vi "Main.vi"() -> ()   [LabVIEW 2011]
panel:
  out "Path":path
  out "Time Stamp":timestamp
  out "Waveform Chart":dbl[](graph)
  out "Error Source Information":string
  in  "stop":bool
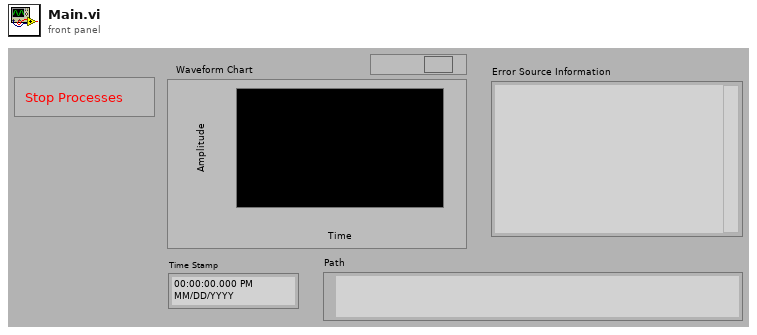
[diagram p1: front panel]
types:
  T1 = cluster{"Data":refnum<user-event>, "Error":refnum<user-event>}
  T2 = cluster{"File Logging":refnum<user-event>, "Error":refnum<user-event>}
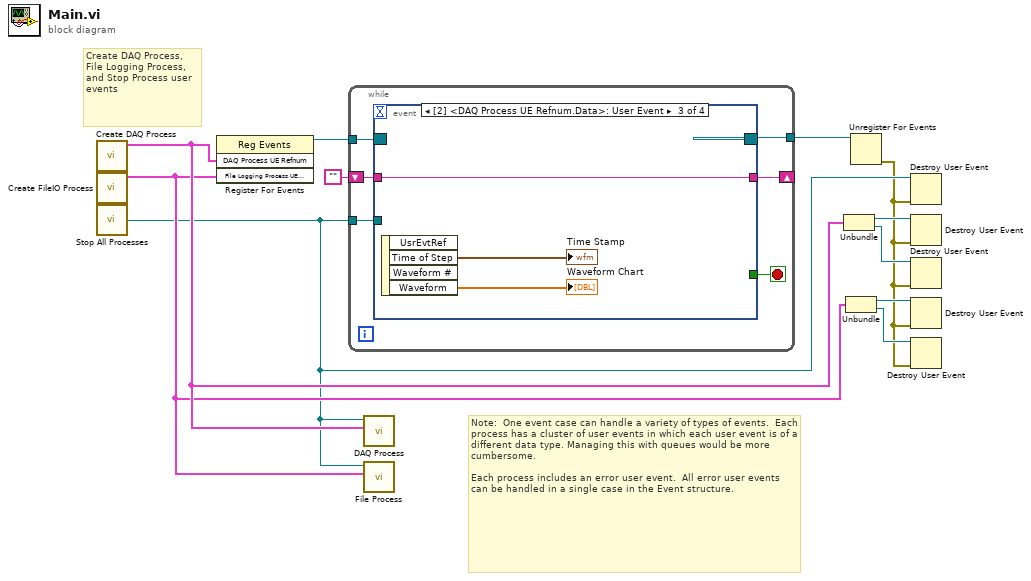
[diagram p0: block diagram]
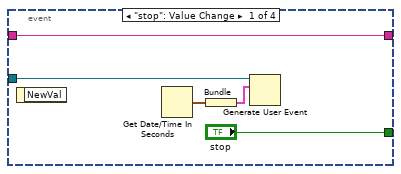
[diagram p2: hidden frame]
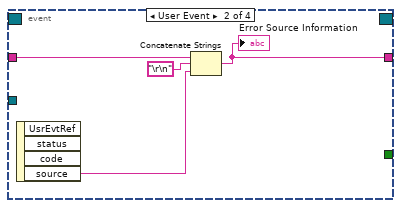
[diagram p3: hidden frame]
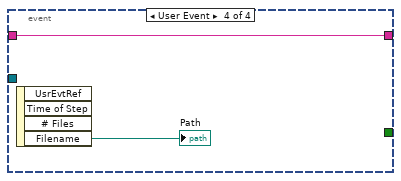
[diagram p4: hidden frame]
diagram:
  # "Create DAQ Process, File Logging Process, and Stop Process user events"
  # "Note:  One event case can handle a variety of types of events.  Each process has a cluster of user events in which each user event is of a different data type. Managing this with queues would be more cumbersome. \n\nEach process includes an error user event.  All error user events can be handled in a single case in the Event structure."
  n1 = call "Create DAQ Process.vi"() -> ("DAQ Process UE Refnum"=w9:T1)  [unwired: 11 in]
  n2 = call "Create FileIO Process.vi"() -> ("File Logging Process UE Refnum"=w3:T2)  [unwired: 11 in]
  n3 = call "Stop All Processes.vi"() -> ("Stop Process"=w2:refnum<user-event>)
  n4 = register-events(w9, w3) -> (reference out=w11:refnum<event-registration>)  [unwired: 2 in, 1 out]
  n5 = while {
    tunnel: w2 -> [w17]
    tunnel: w11 -> [w15]
    tunnel: [w14] -> w10
    shift-right: [w13] -> _
    shift-left: "" -> [w12]
    stop <- w16 stop-if-true
    n6 = event shown="[2] <DAQ Process UE Refnum.Data>: User Event" {
      selector: w15 -> [_ _ _ _]
      dyn-events: [_ _ _ _] -> w14
      timeout: _ -> [_ _ _ _]
      tunnel: w17 -> [w22 _ _ _]
      tunnel: ["stop" _ _ _] -> w16
      tunnel: [w18 w26 w27 w30] -> w13
      tunnel: w12 -> [w18 w25 w27 w30]
      event "stop": Value Change {
        n7 = event-data() -> ()  [unwired: 1 in, 1 out]
        n8 = Get Date/Time In Seconds() -> (seconds since 1Jan1904=w21:timestamp)
        n9 = Bundle("seconds since 1Jan1904"=w21) -> (w20:cluster{"seconds since 1Jan1904":timestamp})  [unwired: 1 in]
        n10 = Generate User Event(user event=w22, event data cluster=w20) -> ()  [unwired: 1 in, 2 out]
      }
      event User Event {
        n11 = event-data() -> ("source"=w24:string)  [unwired: 1 in, 3 out]
        n12 = Concatenate Strings(w25, "\r\n", w24) -> (w26:string)
        "Error Source Information" <- w26
      }
      event User Event {
        n13 = event-data() -> ("Time of Step"=→"Time Stamp":timestamp, "Waveform"=→"Waveform Chart":dbl[])  [unwired: 1 in, 2 out]
      }
      event User Event {
        n14 = event-data() -> ("Filename"=→"Path":path)  [unwired: 1 in, 3 out]
      }
    }
  }
  n15 = call "DAQ Process.vi"("DAQ Process UE Refnum"=w9, "All Stop"=w2) -> ()  [unwired: 10 in]
  n16 = call "File Process.vi"("File Logging Process UE Refnum"=w3, "All Stop"=w2) -> ()  [unwired: 10 in]
  n17 = Unbundle(w9) -> ("Data"=w8:refnum<user-event>, "Error"=w5:refnum<user-event>)
  n18 = Unbundle(w3) -> ("File Logging"=w7:refnum<user-event>, "Error"=w6:refnum<user-event>)
  n19 = Unregister For Events(event registration refnum=w10) -> (error out=w1:errorcluster)  [unwired: 1 in]
  n20 = Destroy User Event(user event=w2, error in=w1) -> ()  [unwired: 1 out]
  n21 = Destroy User Event(user event=w8, error in=w1) -> ()  [unwired: 1 out]
  n22 = Destroy User Event(user event=w5, error in=w1) -> ()  [unwired: 1 out]
  n23 = Destroy User Event(user event=w7, error in=w1) -> ()  [unwired: 1 out]
  n24 = Destroy User Event(user event=w6, error in=w1) -> ()  [unwired: 1 out]
